vi "2_Subscribe.vi"(8 "error in (no error)":errorcluster caption="错误输入（无错误）", 9 "Subscribe":T1, 11 "MQTT_Client_Actor 输入":refnum<class "MQTT_Client_Actor.lvclass">) -> (0 "error out":errorcluster caption="错误输出", 3 "MQTT_Client_Actor 输出":refnum<class "MQTT_Client_Actor.lvclass">)   [LabVIEW 2018, in "MQTT_Client_Actor.lvlib" / "MQTT_Client_Actor.lvclass"]
uses:
  MQTT_Client_Actor.lvclass
  SubscribeClient.ctl
  <vilib>/LabVIEW Open Source Project/MQTT Control Packets/Control Packets/ControlPacket/QualityOfService -- enum.ctl
  MQTT_Client_Actor.lvclass/MQTT_Client_Actor.ctl
  <vilib>/LabVIEW Open Source Project/MQTT Control Packets/Control Packets/ControlPacket/ControlPacket.lvclass
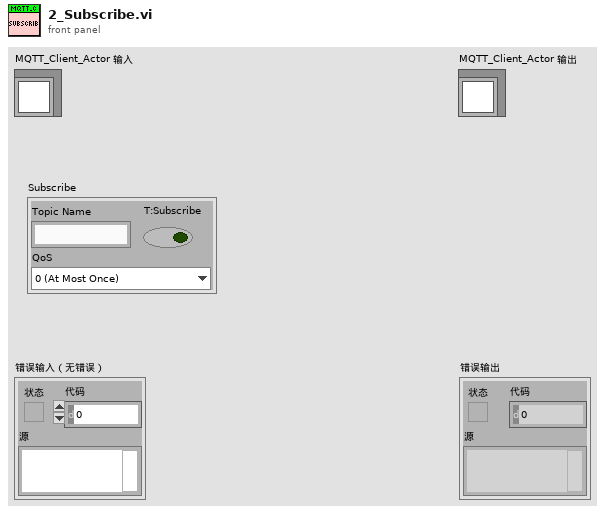
[diagram p1: front panel]
types:
  T1 = typedef "MQTT_Client_Actor.lvlib/MQTT_Client_Actor.lvclass/SubscribeClient.ctl" = cluster{"Topic Name":string, "QoS":T2, "T:Subscribe":bool}
  T2 = typedef "MQTT_Control_Packets.lvlib/ControlPacket.lvclass/QualityOfService -- enum.ctl" = enum16{"0 (At Most Once)", "1 (At Least Once)", "2 (Exactly Once)"}
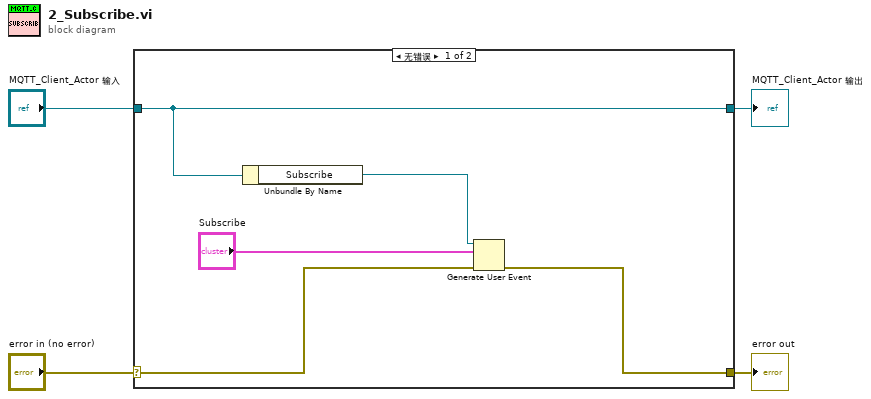
[diagram p0: block diagram]
diagram:
  n1 = case shown="无错误" "error in (no error)" {
    selector: "error in (no error)" -> [w6 w11]
    tunnel: [w5 w11] -> w3
    tunnel: [w9 w10] -> w1
    tunnel: "MQTT_Client_Actor 输入" -> [w9 w10]
    frame No Error {
      n2 = Unbundle By Name(w9) -> ("Subscribe"=w8:refnum<user-event>)
      n3 = Generate User Event(user event=w8, event data cluster="Subscribe", error in=w6) -> (error out=w5:errorcluster)  [unwired: 1 in, 1 out]
    }
    frame Error {
    }
  }
  "error out" <- w3
  "MQTT_Client_Actor 输出" <- w1
